vi "Run Script.vi"(5 "Script Name":string="Clear Well+Lines X", 7 "Main References":T4, 8 "error in (no error)":errorcluster, 9 "Drain X":T2, 10 "Well X":T1, 11 "Bottle X":T3) -> (0 "error out":errorcluster)   [LabVIEW 2018]
uses:
  Main Refs.ctl
  Hardware/Tecan/Pump Config.ctl
  Vacuum Specs.ctl
  Cartridges.ctl
  Cartridge Status.ctl
  Commands.ctl
  Lib/Time/Wells.ctl
  Lib/Time/Bottles.ctl
  Process State.ctl
  Vacuum Test.ctl
  Drain Valve.ctl
  Script Mngr Action.ctl
  Script Mngr Script choice.ctl
  Main Globals.vi
panel:
  # "Tecan Pump"
  # "Vacuum"
  # "General"
  # "Protocol"
  # "Zaber"
  # "NFC Reader 1"
  # "NFC  Reader 2"
  # "NFC Reader 3"
  # "NFC Reader 4"
  # "System"
  # "Cartridge Utitlies"
  # "Wells"
  # "times"
  # "from"
  # "State Machine"
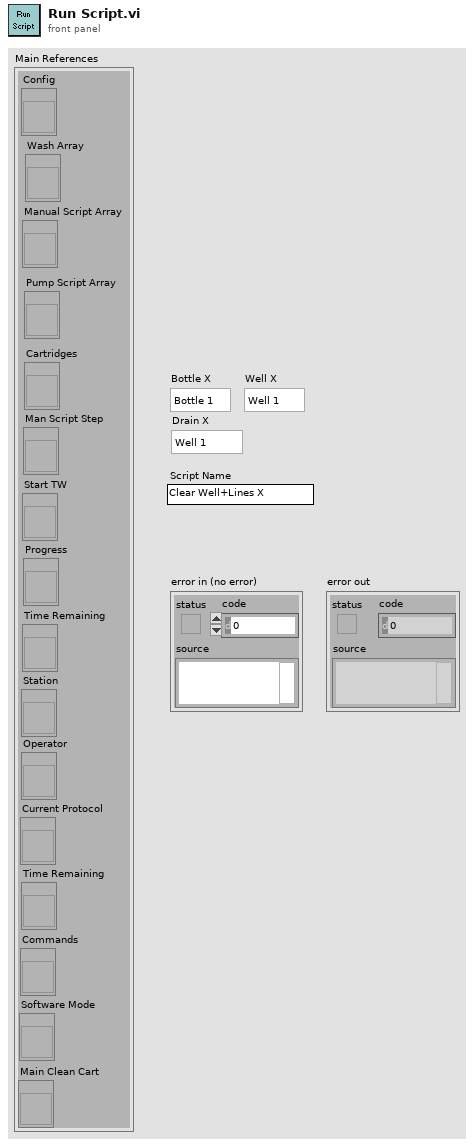
[diagram p1: front panel]
types:
  T1 = typedef "Wells.ctl" = enum16{"Well 1", "Well 2", "Well 3", "Well 4"}
  T2 = typedef "Drain Valve.ctl" = enum16{"Well 1", "Well 2", "Well 3", "Well 4", "Well X"}
  T3 = typedef "Bottles.ctl" = enum16{"Bottle 1", "Bottle 2", "Bottle 3", "H2O", "Waste"}
  T4 = typedef "Main Refs.ctl" = cluster{"Config":refnum<vi>, "Wash Array":refnum<vi>, "Manual Script Array":refnum<vi>, "Pump Script Array":refnum<vi>, "Cartridges":refnum<vi>, "Man Script Step":refnum<vi>, "Start TW":refnum<vi>, "Progress":refnum<vi>, "Time Remaining":refnum<vi>, "Station":refnum<vi>, "Operator":refnum<vi>, "Current Protocol":refnum<vi>, "Time Remaining":refnum<vi>, "Commands":refnum<vi>, "Software Mode":refnum<vi>, "Main Clean Cart":refnum<vi>}
  T5 = typedef "Script Mngr Script choice.ctl" = enum16{"Manual Script", "Pump Script", "Wash Setup"}
  T6 = typedef "Script Mngr Action.ctl" = enum16{"Init", "Run Script", "Load Script", "Save Script", "Close"}
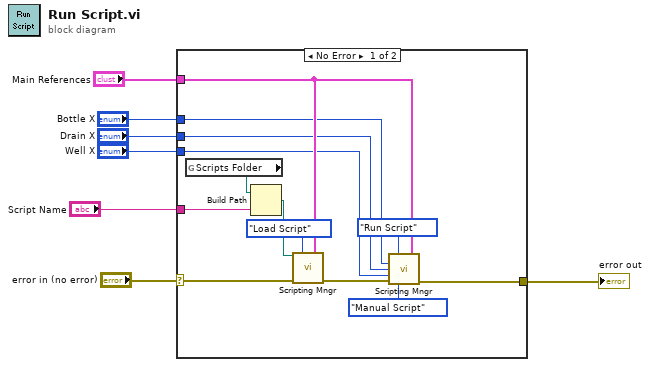
[diagram p0: block diagram]
diagram:
  n1 = case shown="No Error" "error in (no error)" {
    selector: "error in (no error)" -> [w8 w21]
    tunnel: "Script Name" -> [w19 _]
    tunnel: "Main References" -> [w13 _]
    tunnel: [w12 w21] -> w5
    tunnel: "Bottle X" -> [w11 _]
    tunnel: "Drain X" -> [w10 _]
    tunnel: "Well X" -> [w9 _]
    frame No Error {
      n2 = global read "Main Globals.vi" "Scripts Folder"() -> (w18:path)
      n3 = Build Path(base path=w18, name or relative path=w19) -> (appended path=w17:path)
      n4 = call "Scripting Mngr.vi"("Path (dialog)"=w17, "Mngr Action"=Script_Mngr_Action."Load Script", "Main References"=w13, "error in (no error)"=w8) -> ("error out"=w14:errorcluster)  [unwired: 10 in, 1 out]
      n5 = call "Scripting Mngr.vi"("Mngr Action"=Script_Mngr_Action."Run Script", "Main References"=w13, "Bottle X"=w11, "Drain X"=w10, "Well X"=w9, "error in (no error)"=w14, "Script Choice"=Script_Mngr_Script_choice."Manual Script") -> ("error out"=w12:errorcluster)  [unwired: 7 in, 1 out]
    }
    frame Error {
    }
  }
  "error out" <- w5
